vi "3 ch.vi"(8 "error out":errorcluster, 9 "Number of channels":i32, 11 "VISA resource name out":refnum<visa-resource-name>) -> (0 "error out 2":errorcluster, 1 "Means of 12":dbl[](array[numeric]), 2 "Means of 11":dbl[](array[numeric]), 3 "Means of 10":dbl[](array[numeric]), 4 "output array":dbl[](array[numeric]), 5 "VISA resource name out 2":refnum<visa-resource-name>)   [LabVIEW 2015]
uses:
  <instrlib>/Keithley 27XX/Public/Data/Read Multiple Direct.vi
  <instrlib>/Keithley 27XX/Keithley 27XX.lvlib
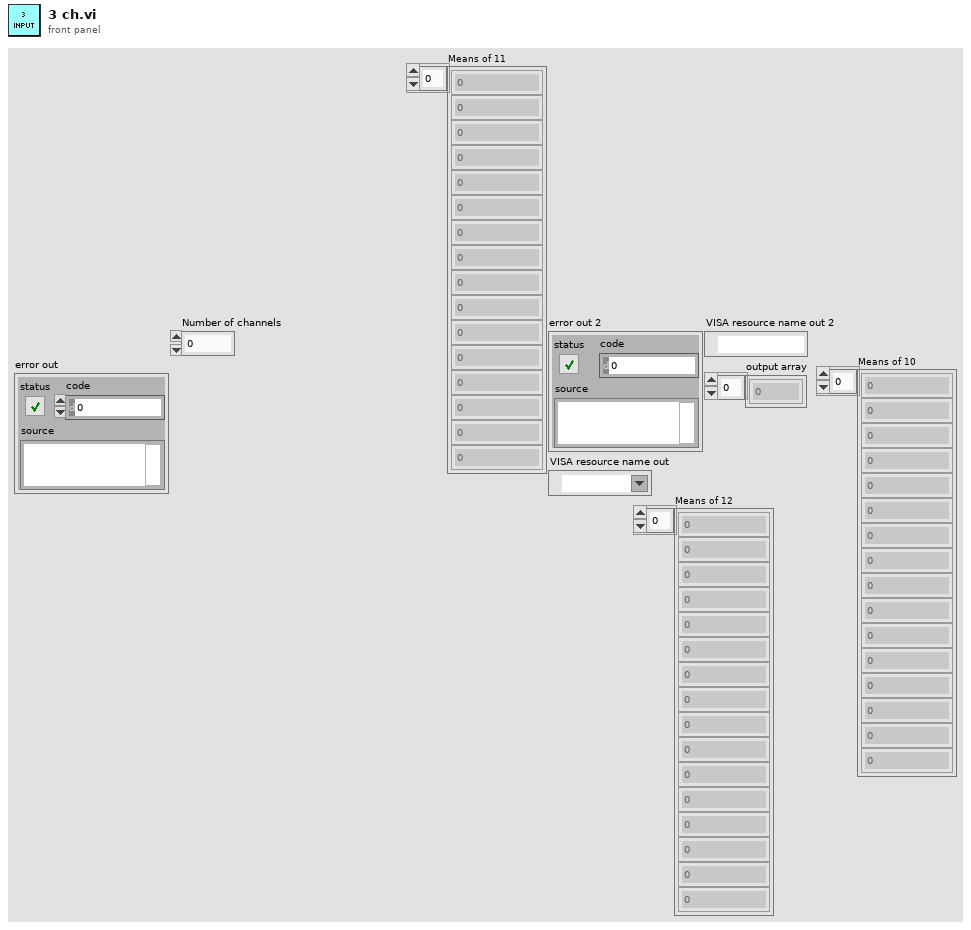
[diagram p1: front panel]
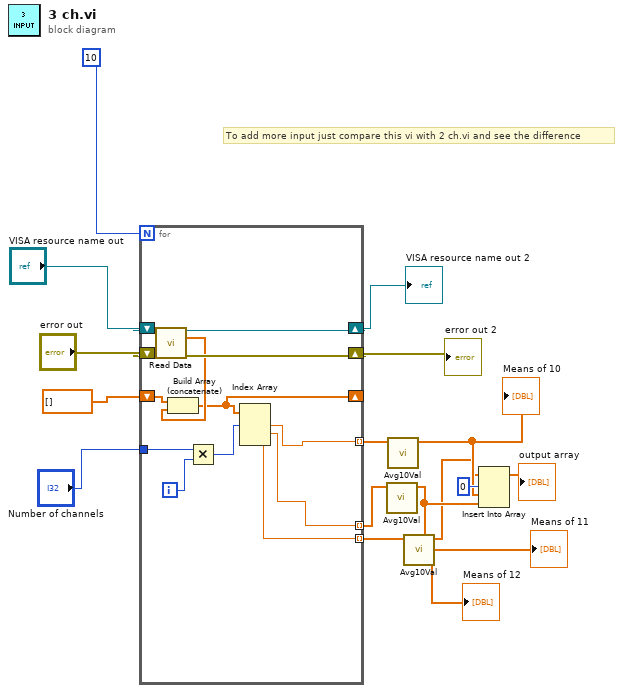
[diagram p0: block diagram]
diagram:
  # "To add more input just compare this vi with 2 ch.vi and see the difference"
  n1 = for {
    N: 10 -> [_]
    shift-right: [w27] -> w14
    shift-left: "VISA resource name out" -> [w26]
    shift-right: [w28] -> w15
    shift-left: "error out" -> [w25]
    shift-right: [w19] -> _
    shift-left: dbl[] [] -> [w24]
    tunnel: "Number of channels" -> [w21]
    tunnel: [w18] -> w10 mode=indexing
    tunnel: [w17] -> w9 mode=indexing
    tunnel: [w16] -> w4 mode=indexing
    i -> [w22]
    n2 = call-poly <instrlib>:"Read Data.vi"("VISA resource name"=w26, "error in (no error)"=w25) -> ("VISA resource name out"=w27:refnum<visa-resource-name>, "Measurement Data"=w23:dbl[], "error out"=w28:errorcluster)  [unwired: 8 in, 3 out]
    n3 = Build Array (concatenate)(w24, w23) -> (w19:dbl[])
    n4 = Multiply(x=w21, y=w22) -> (x*y=w20:i32)
    n5 = Index Array(array=w19, index #1=w20) -> (element #1=w18:dbl, element #2=w17:dbl, element #3=w16:dbl)  [unwired: 2 in]
  }
  "error out 2" <- w15
  "VISA resource name out 2" <- w14
  n6 = call "Avg10Val.vi"("element"=w9) -> ("Means of 10"=w2:dbl[])  [unwired: 10 in]
  "Means of 11" <- w2
  n7 = call "Avg10Val.vi"("element"=w10) -> ("Means of 10"=w3:dbl[])  [unwired: 10 in]
  "Means of 10" <- w3
  n8 = call "Avg10Val.vi"("element"=w4) -> ("Means of 10"=w1:dbl[])  [unwired: 10 in]
  "Means of 12" <- w1
  n9 = Insert Into Array(array=w1, index=0, new element #1=w3, new element #2=w2) -> (→"output array":dbl[])
